vi "guid_generator.vi"() -> (3 "guid":string)   [LabVIEW 2020, in "Caraya.lvlib"]
uses:
  Caraya.lvlib
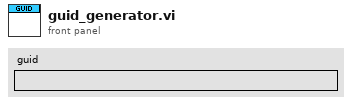
[diagram p1: front panel]
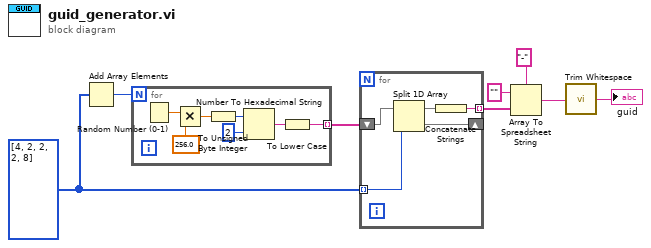
[diagram p0: block diagram]
diagram:
  w6 = i32[] [4, 2, 2, 2, 8]
  n1 = Add Array Elements(numeric array=w6) -> (sum=w8:i32)
  n2 = for {
    N: w8 -> [_]
    tunnel: [w9] -> w7 mode=indexing
    n3 = Random Number (0-1)() -> (number: 0 to 1=w14:dbl)
    n4 = Multiply(x=w14, y=256.0) -> (x*y=w13:dbl)
    n5 = To Unsigned Byte Integer(number=w13) -> (unsigned 8bit integer=w12:u8)
    n6 = Number To Hexadecimal String(1:i16 2 ("width (-)"), 2:w12) -> (0:w10:string)
    n7 = To Lower Case(string=w10) -> (all lower case string=w9:string)
  }
  n8 = for {
    shift-right: [w20] -> _
    shift-left: w7 -> [w19]
    tunnel: w6 -> [w18] mode=indexing
    tunnel: [w16] -> w5 mode=indexing
    n9 = Split 1D Array(array=w19, index=w18) -> (first subarray=w17:string[], second subarray=w20:string[])
    n10 = Concatenate Strings(w17) -> (w16:string)
  }
  n11 = Array To Spreadsheet String(delimiter (Tab)="-", array=w5, 3:"" ("format string")) -> (spreadsheet string=w3:string)
  n12 = call <vilib>:"Trim Whitespace.vi"("string"=w3) -> ("trimmed string"=→"guid":string)  [unwired: 1 in]
